vi "turn negatives to zeroes.vi"(1 "Array in":dbl[](array[numeric])) -> (0 "Array out":dbl[](array[numeric]))   [LabVIEW 2009]
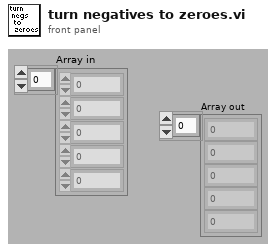
[diagram p1: front panel]
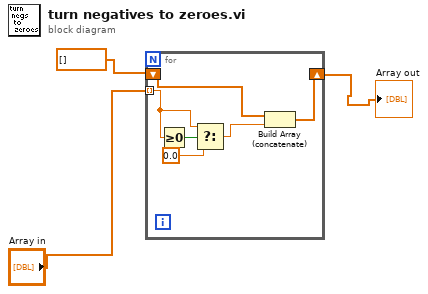
[diagram p0: block diagram]
diagram:
  n1 = for {
    tunnel: "Array in" -> [w6] mode=indexing
    shift-right: [w8] -> w3
    shift-left: dbl[] [] ("array") -> [w9]
    n2 = Greater Or Equal To 0?(x=w6) -> (x >= 0?=w7:bool)
    n3 = Select(t=w6, s=w7, f=0.0) -> (s? t:f=w4:dbl)
    n4 = Build Array (concatenate)(w9, w4) -> (w8:dbl[])
  }
  "Array out" <- w3
